vi "Test V Mode.vi"(8 "error in (no error)":errorcluster, 11 "SR7270 Drivers in":refnum<class "SR7270 Drivers.lvclass">) -> (0 "error out":errorcluster, 3 "SR7270 Drivers out":refnum<class "SR7270 Drivers.lvclass">)   [LabVIEW 2016, in "SR7270 Drivers.lvclass"]
uses:
  SR7270 Drivers.lvclass
  Typedefs/IMODE--enum.ctl
  Typedefs/VMODE--enum.ctl
  <vilib>/addons/_JKI Toolkits/Caraya/classes/Assert/Assert.lvclass
  <vilib>/addons/_JKI Toolkits/Caraya/classes/Test/Test.lvclass
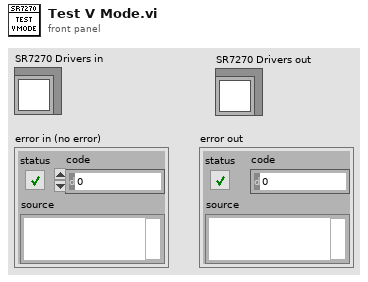
[diagram p1: front panel]
types:
  T1 = typedef "SR7270 Drivers.lvclass/VMODE--enum.ctl" = enum16{"Both Grounded", "A input only", "-B input only", "A-B differential"}
  T2 = typedef "SR7270 Drivers.lvclass/IMODE--enum.ctl" = enum16{"Current Mode Off", "High bandwidth current mode", "Low noise current mode"}
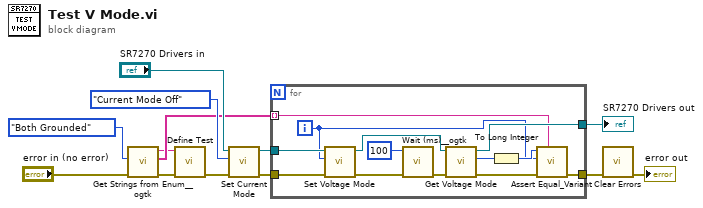
[diagram p0: block diagram]
diagram:
  n1 = call <userlib>:"Get Strings from Enum__ogtk.vi"("error in (no error)"="error in (no error)", "Enum"=VMODE--enum."Both Grounded" ("Voltage Mode")) -> ("error out"=w3:errorcluster, "Enum Strings"=w5:string[], "Enum Name"=w1:string)  [unwired: 6 in, 1 out]
  n2 = call <vilib>:"Define Test.vi"("error in (no error)"=w3, "Label (VI Title)"=w1) -> ("error out"=w13:errorcluster)  [unwired: 9 in]
  n3 = call "Set Current Mode.vi"("error in (no error)"=w13, "Current Mode"=IMODE--enum."Current Mode Off", "SR7270 Drivers in"="SR7270 Drivers in") -> ("error out"=w9:errorcluster, "SR7270 Drivers out"=w12:refnum<class "SR7270 Drivers.lvclass">)  [unwired: 7 in]
  n4 = for {
    tunnel: w12 -> [w25]
    tunnel: w9 -> [w17]
    tunnel: [w23] -> w8
    tunnel: [w22] -> w7
    tunnel: w5 -> [w14] mode=indexing
    i -> [w15]
    n5 = call "Set Voltage Mode.vi"("error in (no error)"=w17, "Voltage Mode"=w15, "SR7270 Drivers in"=w25) -> ("error out"=w19:errorcluster, "SR7270 Drivers out"=w26:refnum<class "SR7270 Drivers.lvclass">)  [unwired: 7 in]
    n6 = call <userlib>:"Wait (ms)__ogtk.vi"("error in (no error)"=w19, "milliseconds to wait"=u32 100) -> ("error out"=w21:errorcluster)  [unwired: 8 in, 1 out]
    n7 = call "Get Voltage Mode.vi"("error in (no error)"=w21, "SR7270 Drivers in"=w26) -> ("error out"=w24:errorcluster, "Voltage Mode"=w18:T1, "SR7270 Drivers out"=w22:refnum<class "SR7270 Drivers.lvclass">)  [unwired: 7 in]
    n8 = To Long Integer(number=w18) -> (32bit integer=w16:i32)
    n9 = call <vilib>:"Assert Equal_Variant.vi"("Label"=w14, "error in (no error)"=w24, "Y"=w15, "X"=w16) -> ("error out"=w23:errorcluster)  [unwired: 7 in]
  }
  "SR7270 Drivers out" <- w7
  n10 = call <vilib>:"Clear Errors.vi"("error in (no error)"=w8) -> ("error out"=→"error out":errorcluster)  [unwired: 5 in, 1 out]
